vi "LinxUartOpen.vi"(8 "Error In":errorcluster, 9 "Baud Rate":u32, 10 "Uart Channel":u8, 11 "LINX Resource":T1) -> (0 "Error Out":errorcluster, 1 "Actual Baud Rate":u32, 3 "LINX Resource":T1)   [LabVIEW 2014, in "LMH-LINX.lvlib" / "Local IO.lvlib"]
uses:
  Local IO.lvlib
  Type Defs/LINX Ref.ctl
  Type Defs/Platform.ctl
  Type Defs/Interface.ctl
  Device/Type Defs/LINX Device Config.ctl
  Device/Type Defs/TCP Config.ctl
  Device/Type Defs/Channels.ctl
  Type Defs/Error Type.ctl
  LMH-LINX.lvlib
  liblinxdevice.dll
  <vilib>/Instr/_visa.llb/VISA Configure Serial Port (Instr).vi
  <vilib>/MakerHub/LINX/Private/Type Defs/Channel FGV States.ctl
  Device/Device.lvlib
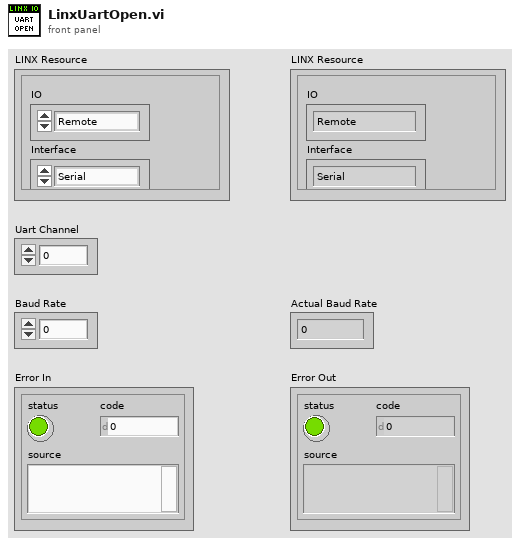
[diagram p1: front panel]
types:
  T1 = typedef "LMH-LINX.lvlib/LINX Ref.ctl" = cluster{"IO":T2, "Interface":T3, "LINX Device Config":T4}
  T2 = typedef "LMH-LINX.lvlib/Platform.ctl" = enum16{"Remote", "Local"}
  T3 = typedef "LMH-LINX.lvlib/Interface.ctl" = enum16{"Serial", "TCP"}
  T4 = typedef "LMH-LINX.lvlib/Device.lvlib/LINX Device Config.ctl" = cluster{"Interface":T3, "COM Port":refnum<visa-resource-name>, "TCP Configuration":T5, "Device Family":u8, "Device ID":u8, "Device Name":string, "TCP Ref":refnum<k5>, "Channels":T6}
  T5 = typedef "LMH-LINX.lvlib/Device.lvlib/TCP Config.ctl" = cluster{"IP Address":string, "Port":u16}
  T6 = typedef "LMH-LINX.lvlib/Channels.ctl" = cluster{"DI":u8[], "DO":u8[], "AI":u8[], "AO":u8[], "PWM":u8[], "QE":u8[], "UART":u8[], "I2C 2":u8[], "SPI":u8[], "CAN":u8[], "Servo":u8[], "AI Ref (V)":dbl, "AI Resolution (Bits)":u8, "AO Ref (V)":dbl, "AO Resolution (Bits)":u8}
  T7 = typedef "LMH-LINX.lvlib/Error Type.ctl" = enum16{"Unknown", "Timeout", "Corrupt Return Packet", "Unable To Connect", "Command Not Supported", "Channel DNE", "Invalid COM Config", "Firmware Version Mismatch", "myRIO Support", "CMD Specific Error", "Local IO Not Supported"}
  T8 = typedef "LMH-LINX.lvlib/Channel FGV States.ctl" = enum16{"Initialize", "Get", "Set"}
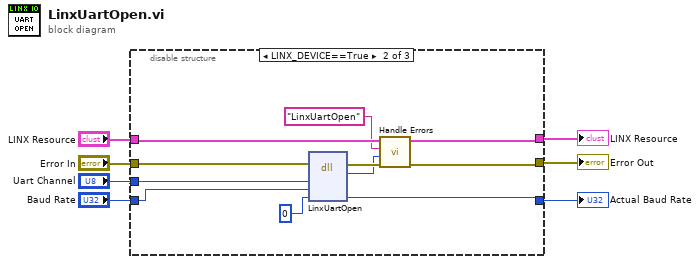
[diagram p0: block diagram]
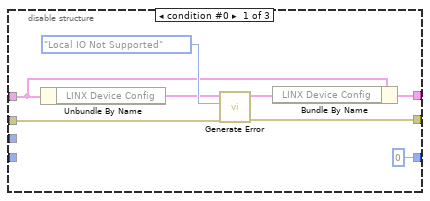
[diagram p2: hidden frame]
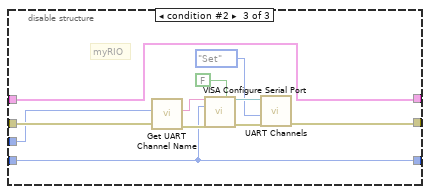
[diagram p3: hidden frame]
diagram:
  n1 = disable-structure shown="LINX_DEVICE==True" {
    disable-tunnel: [w9 w18 w30] -> w6
    disable-tunnel: "LINX Resource" -> [w11 w19 w30]
    disable-tunnel: "Error In" -> [w14 w26 w29]
    disable-tunnel: [w13 w20 w31] -> w7
    disable-tunnel: [u32 0 ("Baud Rate") w25 w27] -> w5
    disable-tunnel: "Uart Channel" -> [_ w23 w28]
    disable-tunnel: "Baud Rate" -> [_ w22 w27]
    frame condition #0 {
      n2 = Unbundle By Name(w11) -> ("LINX Device Config"=w12:T4)
      n3 = call "Generate Error.vi"("Error In"=w14, "Error Type"=Error_Type."Local IO Not Supported", "LINX Device Config"=w12) -> ("Error Out"=w13:errorcluster, "Dup LINX Device Config"=w10:T4)  [unwired: 7 in]
      n4 = Bundle By Name(cluster=w11, "LINX Device Config"=w10) -> (w9:T1)
    }
    frame condition #1 (active) {
      n5 = dll-call lib="liblinxdevice.*" fn="LinxUartOpen"(error in=w26, "channel"=w23, "baudRate"=w22, "actualBaud"=u32 0) -> (error out=w21:errorcluster, "status"=w16:i32, "actualBaud"=w25:u32)  [unwired: 4 in, 1 out]
      n6 = call "Handle Errors.vi"("Error In"=w21, "LinxStatus"=w16, "Function Name"="LinxUartOpen", "LINX Resource"=w19) -> ("Error Out"=w20:errorcluster, "LINX Resource"=w18:T1)  [unwired: 6 in]
    }
    frame condition #2 {
      # "myRIO"
      n7 = call <vilib>:"Get UART Channel Name.vi"("Error In"=w29, "UART Channel"=w28) -> ("Error Out"=w33:errorcluster, "UART Channel"=w34:string)  [unwired: 8 in]
      n8 = call-poly "VISA Configure Serial Port"("VISA resource name"=w34, "Enable Termination\nChar (T)"=FALSE ("Enable Termination\nChar (T)"), "baud rate (9600)"=w27, "error in (no error)"=w33) -> ("VISA resource name out"=w37:refnum<visa-resource-name>, "error out"=w36:errorcluster)  [unwired: 10 in]
      n9 = call <vilib>:"UART Channels.vi"("Error In"=w36, "Channel State"=Channel_FGV_States."Set", "UART Channel"=w37) -> ("Error Out"=w31:errorcluster)  [unwired: 7 in, 1 out]
    }
  }
  "LINX Resource" <- w6
  "Actual Baud Rate" <- w5
  "Error Out" <- w7
